vi "Save.vi"(8 "error in":errorcluster, 10 "file path":path, 11 "repository in":refnum<class "NISE_CEF_HierarchyRepo.lvclass">) -> (0 "error out":errorcluster, 3 "repository out":refnum<class "NISE_CEF_HierarchyRepo.lvclass">)   [LabVIEW 2013, in "NISE_CEF_HierarchyRepo.lvclass"]
doc: "Stores repo information to file. It could save in multiple files or formats at the same time. File versioning is suggested."
uses:
  NISE_CEF_HierarchyRepo.lvclass
  NISE_CEF_HierarchyRepo.lvclass/NISE_CEF_HierarchyRepo.ctl
  tree serializer/NISE_CEF_TreeSerializer.lvlib
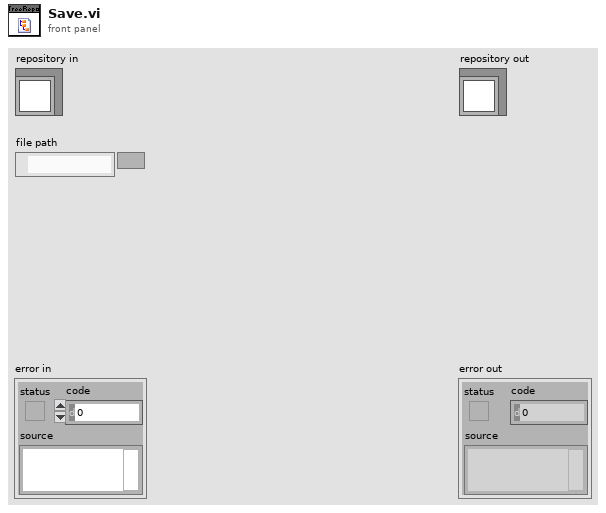
[diagram p1: front panel]
types:
  T1 = typedef "NISE_CEF_TreeSerializer.lvlib/memory hierarchy.ctl" = cluster{"root":string, "hierarchy":T2[], "instance data":refnum<class "NISE_CEF_serializable configuration.lvclass">[]}
  T2 = typedef "NISE_CEF_TreeSerializer.lvlib/hierarchy element.ctl" = cluster{"current node":string, "children":string[]}
  T3 = typedef "NISE_CEF_TreeSerializer.lvlib/file data format.ctl" = cluster{"root":string, "hierarchy":T2[], "instance data":T4[]}
  T4 = typedef "NISE_CEF_TreeSerializer.lvlib/instance data.ctl" = cluster{"ID":string, "Alias":string, "class":string, "version":string, "data":string}
  T5 = typedef "NISE_CEF_TreeSerializer.lvlib/base file format.ctl" = cluster{"version":string, "data":string}
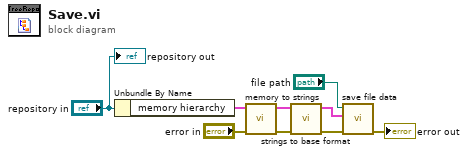
[diagram p0: block diagram]
diagram:
  n1 = Unbundle By Name("repository in") -> ("memory hierarchy"=w4:T1)
  n2 = call "memory to strings.vi"("error in"="error in", "memory hierarchy"=w4) -> ("error out"=w2:errorcluster, "1.0.0"=w3:T3)  [unwired: 8 in]
  n3 = call "strings to base format.vi"("error in"=w2, "1.0.0"=w3) -> ("error out"=w6:errorcluster, "format"=w5:T5)  [unwired: 8 in]
  n4 = call "save file data.vi"("error in"=w6, "format"=w5, "Path"="file path") -> ("error out"=→"error out":errorcluster)  [unwired: 8 in]
  "repository out" <- "repository in"
